vi "DAQmx Create Channel (AI-Force-Bridge-Two-Point-Linear).vi"(0 "task in":refnum<k21>, 1 "maximum value":dbl=100.0 format="%0.2f", 2 "minimum value":dbl=-100.0 format="%0.2f", 3 "bridge information":T1={"bridge configuration"=10182, "voltage excitation source"=10200, "voltage excitation value"=2.5, "nominal bridge resistance"=350.0} {"voltage excitation source" items=["Internal"=10200, "External"=10167]; "bridge configuration" items=["Full Bridge"=10182, "Half Bridge"=10187, "Quarter Bridge"=10270]}, 5 "physical channels":tag, 7 "name to assign":string, 9 "units":i32(ring)=15876 items=["Newtons"=15875, "Pounds"=15876, "kgf"=15877, "From Custom Scale"=10065], 11 "error in":errorcluster, 12 "custom scale name":tag, 14 "scaling information":T2={"first electrical value"=0.0, "second electrical value"=2.0, "electrical units"=15897, "first physical value"=0.0, "second physical value"=100.0, "physical units"=15876} {"physical units" items=["Newtons"=15875, "Pounds"=15876, "kgf"=15877]; "electrical units" items=["Volts/Volt"=15896, "mVolts/Volt"=15897]}) -> (4 "task out":refnum<k21>, 15 "error out":errorcluster)   [LabVIEW 2018]
doc: "Creates channel(s) that use a Wheatstone bridge to measure force or load. Use this instance with sensors whose specifications do not provide a polynomial for scaling or a table of electrical and physical values. When you use this scaling type, NI-DAQmx uses two points of electrical and physical values to calculate the slope and y-intercept of a linear equation and uses that equation to scale electrical values to physical values."
uses:
  nilvaiu.dll
panel:
  # "input limits"
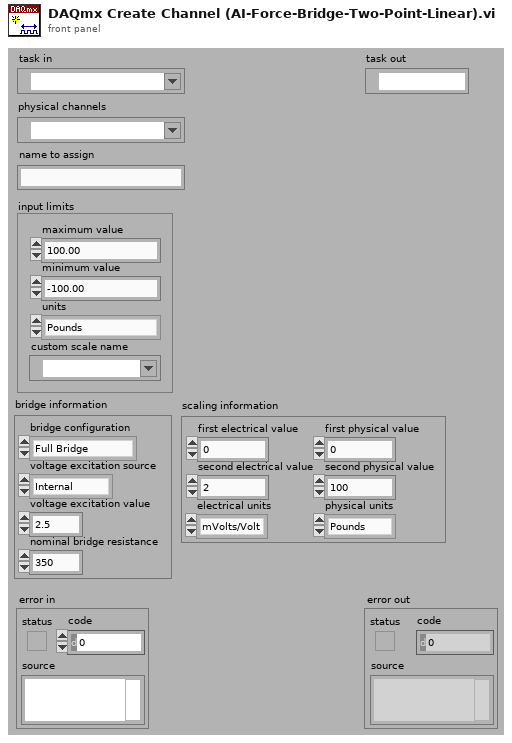
[diagram p1: front panel]
types:
  T1 = cluster{"bridge configuration":i32, "voltage excitation source":i32, "voltage excitation value":dbl, "nominal bridge resistance":dbl}
  T2 = cluster{"first electrical value":dbl, "second electrical value":dbl, "electrical units":i32, "first physical value":dbl, "second physical value":dbl, "physical units":i32}
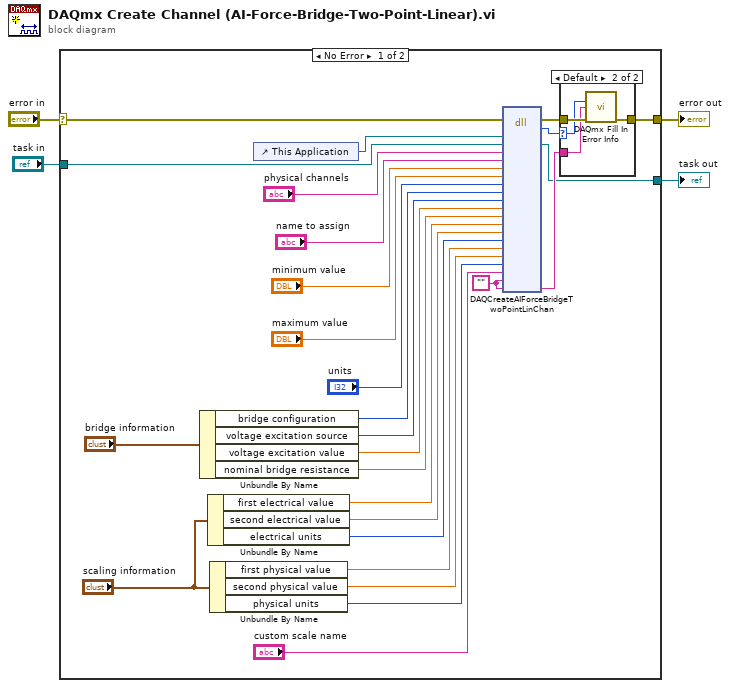
[diagram p0: block diagram]
diagram:
  n1 = case shown="No Error" "error in" {
    selector: "error in" -> [w22 w37]
    tunnel: [w26 w37] -> w4
    tunnel: "task in" -> [w21 w38]
    tunnel: [w6 w38] -> w1
    frame No Error {
      w5 = ""
      n2 = Unbundle By Name("bridge information") -> ("bridge configuration"=w10:i32, "voltage excitation source"=w9:i32, "voltage excitation value"=w8:dbl, "nominal bridge resistance"=w7:dbl)
      n3 = Unbundle By Name("scaling information") -> ("first electrical value"=w16:dbl, "second electrical value"=w15:dbl, "electrical units"=w14:i32)
      n4 = Unbundle By Name("scaling information") -> ("first physical value"=w13:dbl, "second physical value"=w12:dbl, "physical units"=w11:i32)
      n5 = control-ref of="This Application"() -> (w20:refnum<vi>)
      n6 = dll-call lib="nilvaiu.*" fn="DAQCreateAIForceBridgeTwoPointLinChan"(error in=w22, "lvAppRef"=w20, "refObjPtr"=w21, "physicalChannelName"="physical channels", "channelNameIn"="name to assign", "minVal"="minimum value", "maxVal"="maximum value", "units"="units", "bridgeConfig"=w10, "voltageExcitSource"=w9, "voltageExcitVal"=w8, "nominalBridgeResistance"=w7, "firstElectricalValue"=w16, "secondElectricalValue"=w15, "electricalUnits"=w14, "firstPhysicalValue"=w13, "secondPhysicalValue"=w12, "physicalUnits"=w11, "customScaleName"="custom scale name", "channelNamesOut"=w5, "extendedErrorInfo"=w5) -> (error out=w27:errorcluster, "return type"=w29:i32, "refObjPtr"=w6:refnum<k21>, "extendedErrorInfo"=w28:string)  [unwired: 20 in, 1 out]
      n7 = case shown="Default" w29 {
        selector: w29 -> [_ w34]
        tunnel: w27 -> [w32 w36]
        tunnel: [w32 w35] -> w26
        tunnel: w28 -> [_ w33]
        frame 0 {
        }
        frame Default {
          n8 = call "DAQmx Fill In Error Info.vi"("status code"=w34, "extended error info"=w33, "error in"=w36) -> ("error out"=w35:errorcluster)  [unwired: 1 in, 11 out]
        }
      }
    }
    frame Error {
    }
  }
  "error out" <- w4
  "task out" <- w1
